vi "Example Callback.vi"() -> ()   [LabVIEW 2010]
uses:
  C:/tf/play/labview/Tinkerforge.dll
  Tinkerforge.dll
panel:
  in  "stop":bool
  out "illuminance (Lux)":sgl format="%#_13g"
  in  "uid":string="amb"
  in  "port":i32=4223
  in  "host":string="localhost"
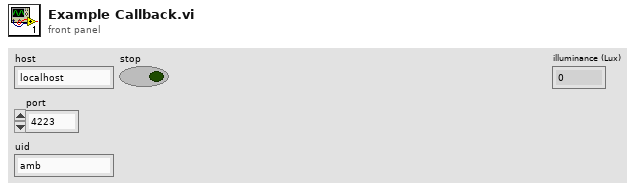
[diagram p1: front panel]
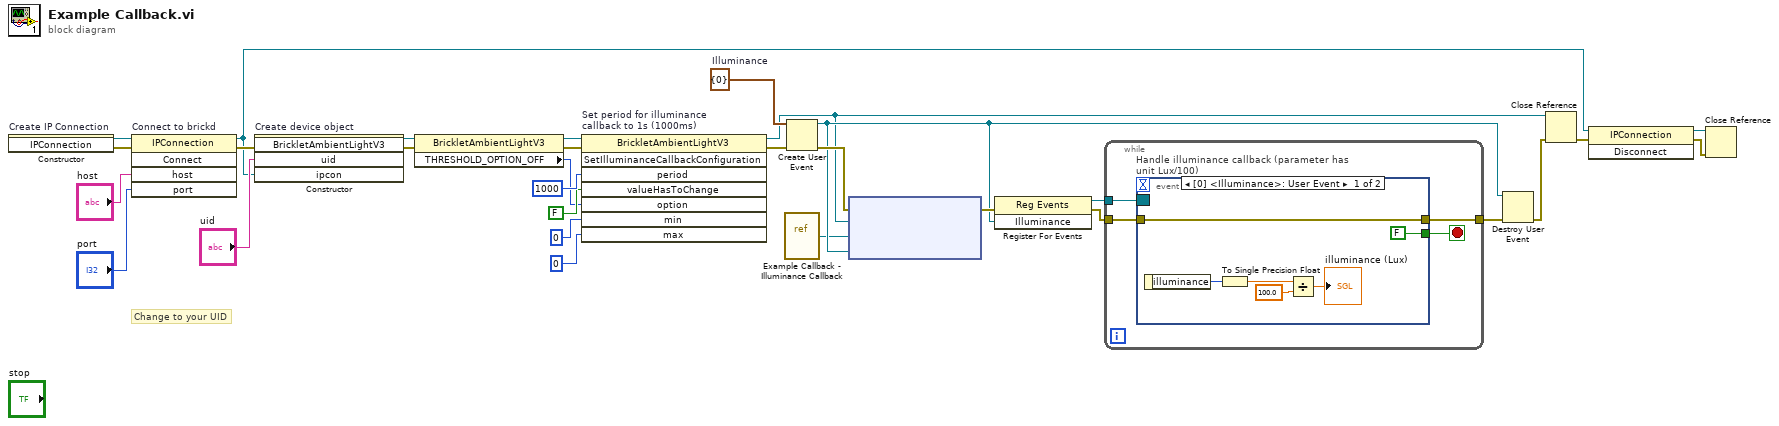
[diagram p0: block diagram]
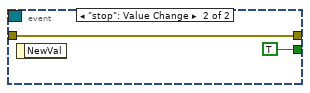
[diagram p2: hidden frame]
diagram:
  w14 = cluster{"illuminance":i64} {"illuminance"=0}  # Illuminance
  # "Change to your UID"
  n1 = constructor on="Create IP Connection" class="IPConnection"() -> (reference out=w30:refnum<k24>, error out=w10:errorcluster)  [unwired: 3 in, 1 out]
  n2 = invoke on="Connect to brickd" class="IPConnection" method="Connect"(reference=w30, error in=w10, "host"="host", "port"="port") -> (reference out=w23:refnum<k24>, error out=w26:errorcluster)  [unwired: 1 in, 3 out]
  n3 = constructor on="Create device object" class="BrickletAmbientLightV3"(error in=w26, "uid"="uid", "ipcon"=w23) -> (reference out=w4:refnum<k24>, error out=w7:errorcluster)  [unwired: 2 in, 3 out]
  n4 = property class="BrickletAmbientLightV3"(reference=w4, error in=w7) -> (reference out=w5:refnum<k24>, error out=w6:errorcluster, "THRESHOLD_OPTION_OFF"=w3:u16)
  n5 = invoke on="Set period for illuminance\ncallback to 1s (1000ms)" class="BrickletAmbientLightV3" method="SetIlluminanceCallbackConfiguration"(reference=w5, error in=w6, "period"=i64 1000, "valueHasToChange"=FALSE, "option"=w3, "min"=i64 0, "max"=i64 0) -> (reference out=w12:refnum<k24>, error out=w13:errorcluster)  [unwired: 1 in, 6 out]
  n6 = vi-ref "Example Callback - Illuminance Callback.vi"() -> ("vi reference"=w9:refnum<vi>)
  n7 = Create User Event(user event datatype=w14, error in=w13) -> (user event=w16:refnum<user-event>, error out=w21:errorcluster)
  n8 = node ("Register Event Callback")(w21, w12, w9, w16) -> (w20:errorcluster)  [unwired: 1 in, 1 out]
  n9 = register-events(error in=w20, w16) -> (reference out=w19:refnum<event-registration>, error out=w17:errorcluster)  [unwired: 1 in]
  n10 = while {
    tunnel: w19 -> [w34]
    tunnel: [w33] -> w18
    tunnel: w17 -> [w32]
    stop <- w31 stop-if-true
    n11 = event "Handle illuminance callback (parameter has unit Lux/100)" shown="[0] <Illuminance>: User Event" {
      selector: w34 -> [_ _]
      dyn-events: _ -> [_ _]
      timeout: _ -> [_ _]
      tunnel: [w37 w41] -> w33
      tunnel: w32 -> [w37 w41]
      tunnel: [FALSE TRUE] -> w31
      event User Event {
        n12 = event-data() -> ("illuminance"=w38:i64)  [unwired: 1 in]
        n13 = To Single Precision Float(number=w38) -> (single precision float=w39:sgl)
        n14 = Divide(x=w39, y=sgl 100.0) -> (x/y=→"illuminance (Lux)":sgl)
      }
      event "stop": Value Change {
        n15 = event-data() -> ()  [unwired: 1 in, 1 out]
      }
    }
  }
  n16 = Destroy User Event(user event=w16, error in=w18) -> (error out=w15:errorcluster)
  n17 = Close Reference(reference=w12, error in (no error)=w15) -> (error out=w25:errorcluster)
  n18 = invoke class="IPConnection" method="Disconnect"(reference=w23, error in=w25) -> (reference out=w22:refnum<k24>, error out=w24:errorcluster)  [unwired: 1 in, 1 out]
  n19 = Close Reference(reference=w22, error in (no error)=w24) -> ()  [unwired: 1 out]
